vi "c ctre phoenix report error.vi"(5 "callStack":string, 6 "location":string, 7 "details":string, 8 "error in (no error)":errorcluster, 9 "isLVCode":i32, 10 "errorCode":i32, 11 "isError":i32) -> (0 "error out":errorcluster)   [LabVIEW 2020, in "CTRE_PhoenixTools.lvlib"]
doc: "CTREXPORT void c_ctre_phoenix_report_error(int isError, int32_t errorCode, int isLVCode, const char *details,\n const char *location, const char *callStack);"
uses:
  CTRE_PhoenixTools.lvlib
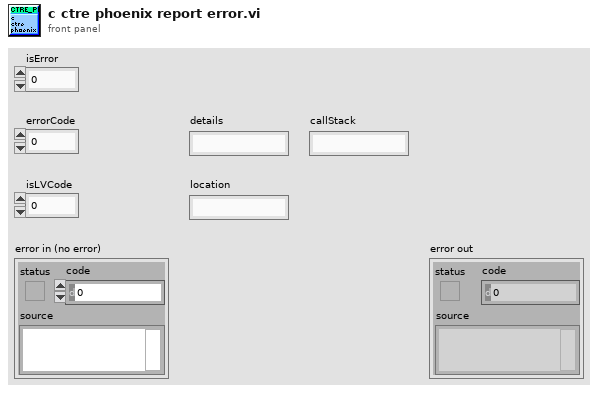
[diagram p1: front panel]
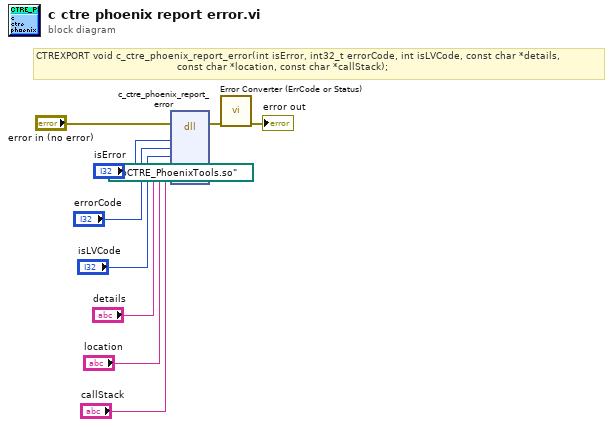
[diagram p0: block diagram]
diagram:
  # "CTREXPORT void c_ctre_phoenix_report_error(int isError, int32_t errorCode, int isLVCode, const char *details,\n                                               const char *location, const char *callStack);"
  n1 = dll-call lib="?" fn="c_ctre_phoenix_report_error"(path in=path "libCTRE_PhoenixTools.so", error in="error in (no error)", "isError"="isError", "errorCode"="errorCode", "isLVCode"="isLVCode", "details"="details", "location"="location", "callStack"="callStack") -> (error out=w3:errorcluster)  [unwired: 8 in, 1 out]
  n2 = call "Error Converter (ErrCode or Status).vi"("error in (no error)"=w3) -> ("error out"=→"error out":errorcluster)  [unwired: 10 in]
